vi "III_V_Layer_v23.vi"(2 "Debug Mode":bool, 3 "Elapsed Time(s)":dbl, 4 "State":enum16{"Edit", "Start", "Run", "End", "Idle"}(ring), 5 "Argument List In":string[](array[string])) -> (0 "Status Out":string, 1 "Argument List Out":string[](array[string]))   [LabVIEW 2011]
uses:
  high_level_proc/source_dilution.ctl
  high_level_proc/source_noDilution.ctl
panel:
  in  "run_time":dbl caption="Run Time (s)"
  in  "total_time":dbl
  in  "Ring":u16(ring)
  out "source array":refnum<vi>[](array[refnum])
  in  "Zn_bubbler":T1={"Dilution"=FALSE, "Calculated"=0, "MFC1 flow"=0.0, "MFC2 flow"=10.0, "MFC3 flow"=100.0, "Main"={"Flow"=0.0, "Prep"=FALSE, "Run"=FALSE, "Active"=FALSE, "Name"="Zn"}} caption="Al" {"Main"."Flow" format="%.2f"; "MFC1 flow" format="%.4f"; "MFC3 flow" format="%.1f"; "MFC2 flow" format="%.2f"; "Calculated" items=["Flow", "MFC1", "MFC2", "MFC3"]}
  in  "Al_bubbler":T2={"Flow"=0.0, "Prep"=FALSE, "Run"=FALSE, "Active"=FALSE, "Name"="Al"} caption="Al" {"Flow" format="%.2f"}
  in  "Se_bubbler":T1={"Dilution"=FALSE, "Calculated"=0, "MFC1 flow"=0.0, "MFC2 flow"=10.0, "MFC3 flow"=100.0, "Main"={"Flow"=0.0, "Prep"=FALSE, "Run"=FALSE, "Active"=FALSE, "Name"="Se"}} caption="Al" {"Main"."Flow" format="%.2f"; "MFC1 flow" format="%.4f"; "MFC3 flow" format="%.1f"; "MFC2 flow" format="%.2f"; "Calculated" items=["Flow", "MFC1", "MFC2", "MFC3"]}
  in  "P_bubbler":T2={"Flow"=0.0, "Prep"=FALSE, "Run"=FALSE, "Active"=FALSE, "Name"="P liq"} caption="Al" {"Flow" format="%.2f"}
  in  "As_gas":T2={"Flow"=0.0, "Prep"=FALSE, "Run"=FALSE, "Active"=FALSE, "Name"="As gas"} caption="Al" {"Flow" format="%.2f"}
  in  "P_gas":T2={"Flow"=0.0, "Prep"=FALSE, "Run"=FALSE, "Active"=FALSE, "Name"="P gas"} caption="Al" {"Flow" format="%.2f"}
  in  "In_bubbler":T2={"Flow"=0.0, "Prep"=FALSE, "Run"=FALSE, "Active"=FALSE, "Name"="In"} caption="Al" {"Flow" format="%.2f"}
  in  "Ga_bubbler":T1={"Dilution"=FALSE, "Calculated"=0, "MFC1 flow"=0.0, "MFC2 flow"=10.0, "MFC3 flow"=100.0, "Main"={"Flow"=0.0, "Prep"=FALSE, "Run"=FALSE, "Active"=FALSE, "Name"="Ga"}} caption="Al" {"Main"."Flow" format="%.2f"; "MFC1 flow" format="%.4f"; "MFC3 flow" format="%.1f"; "MFC2 flow" format="%.2f"; "Calculated" items=["Flow", "MFC1", "MFC2", "MFC3"]}
  out "prep_done":bool
  out "run started":bool
  out "first":bool=TRUE
  out "is OK?":bool
  in  "prep_time":dbl caption="Pre-Run Time (s)"
  in  "Cancel":bool
  in  "OK":bool
  # "s"
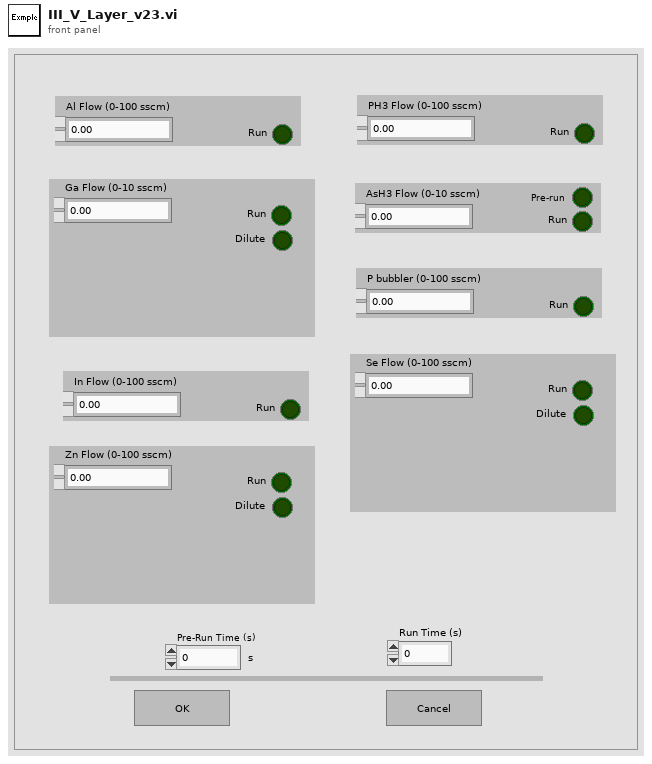
[diagram p1: front panel]
types:
  T1 = typedef "source_dilution.ctl" = cluster{"Dilution":bool, "Calculated":u16, "MFC1 flow":dbl, "MFC2 flow":dbl, "MFC3 flow":dbl, "Main":T2}
  T2 = typedef "source_noDilution.ctl" = cluster{"Flow":dbl, "Prep":bool, "Run":bool, "Active":bool, "Name":string}
  T3 = enum32{"Invalid", "Default", "Floating", "Floating/Auto-Hide", "Modal"}
  T4 = enum16{"Discrete", "Continuous", "Instantaneous", "Finite"}
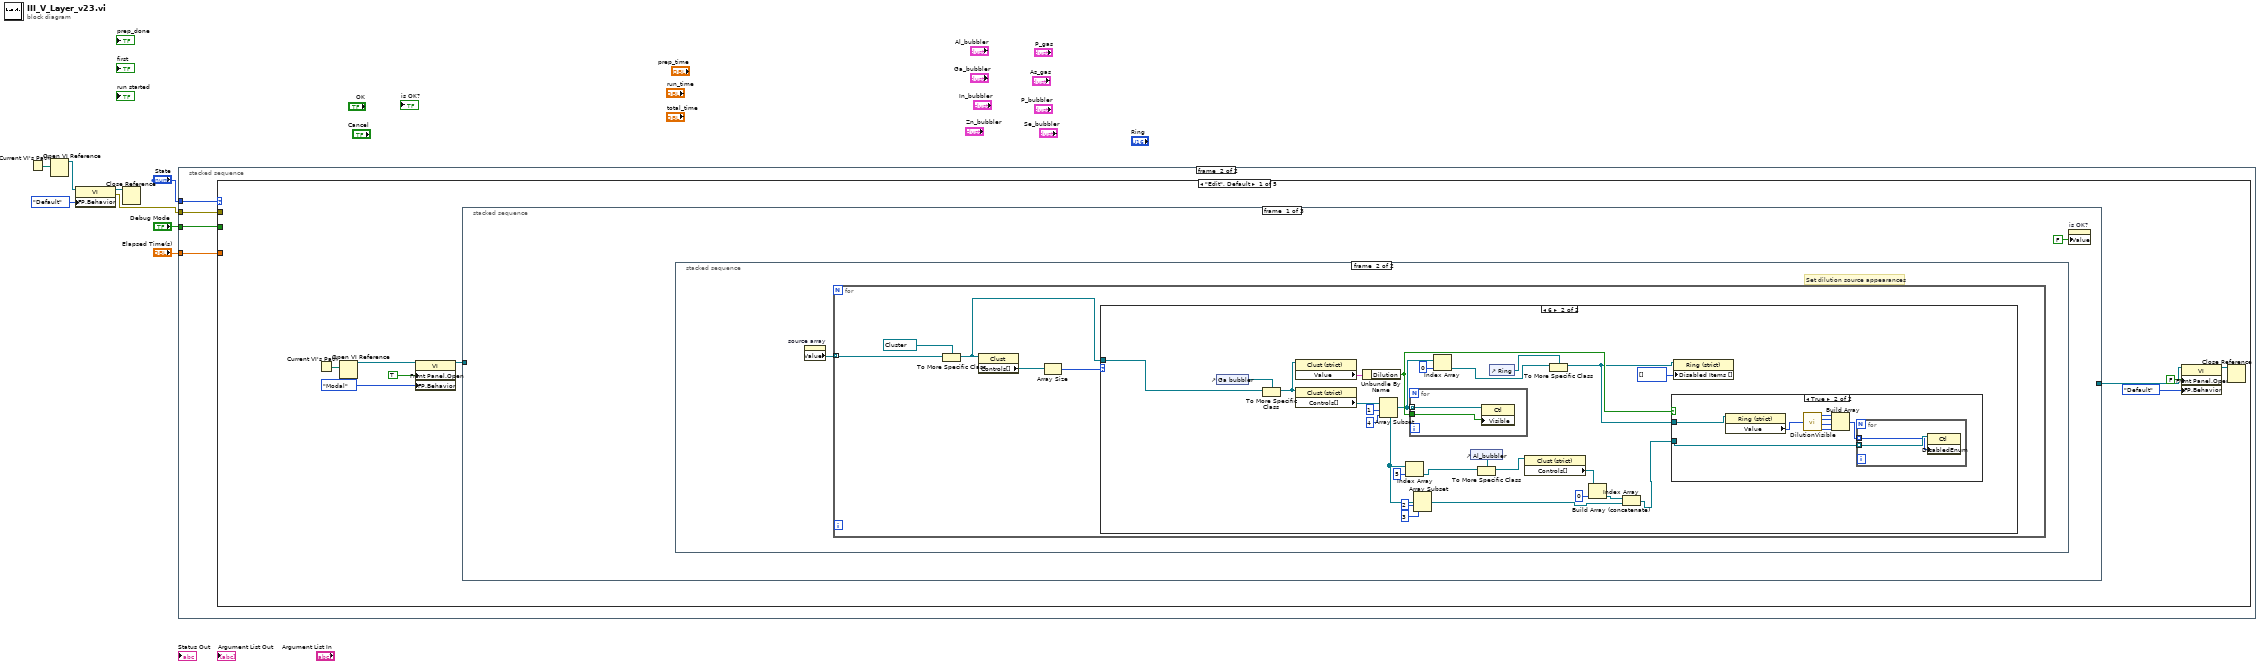
[diagram p0: block diagram]
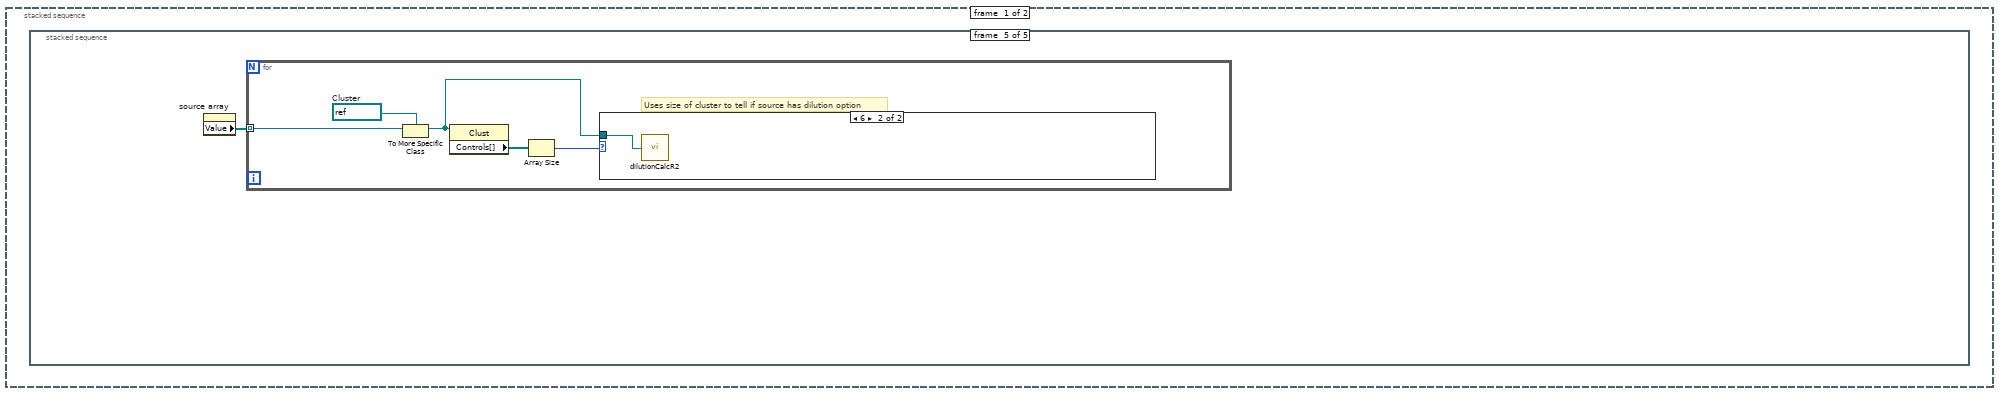
[diagram p2: hidden frame]
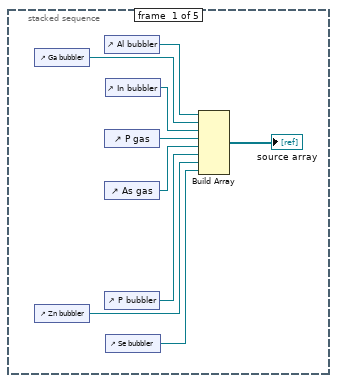
[diagram p3: hidden frame]
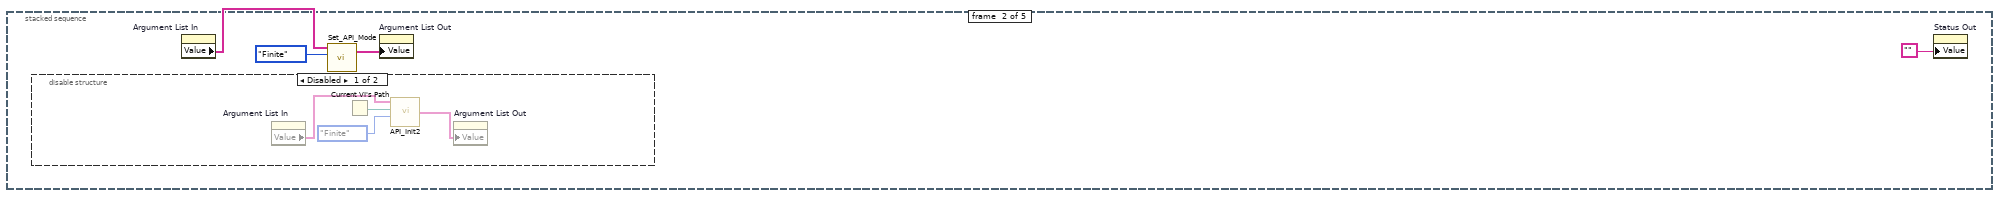
[diagram p4: hidden frame]
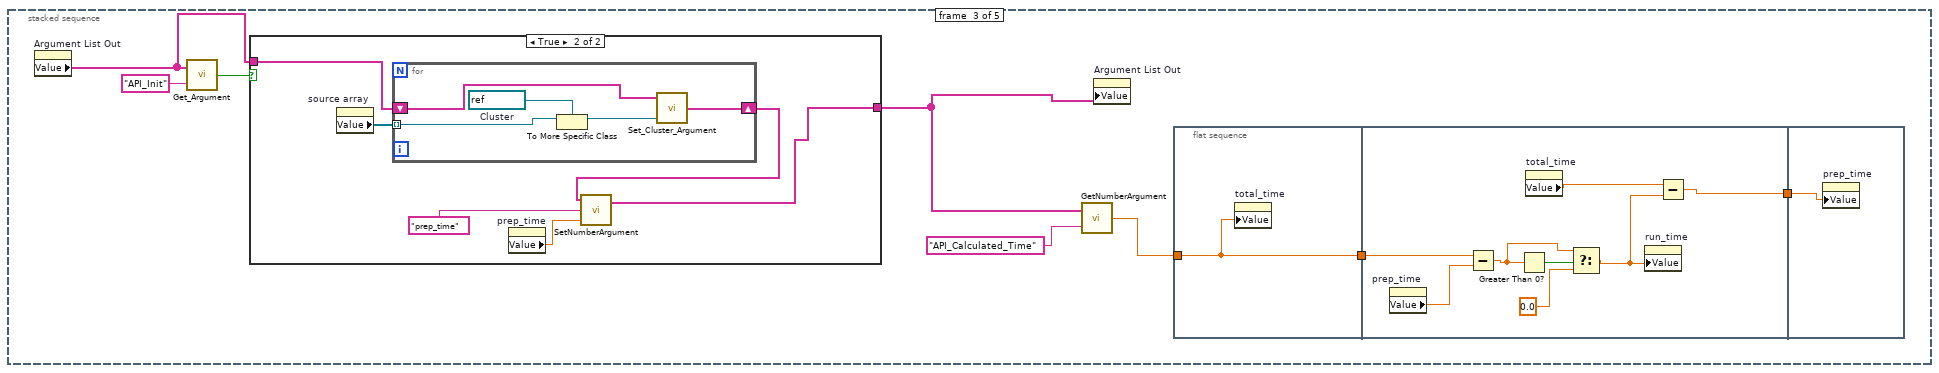
[diagram p6: hidden frame]
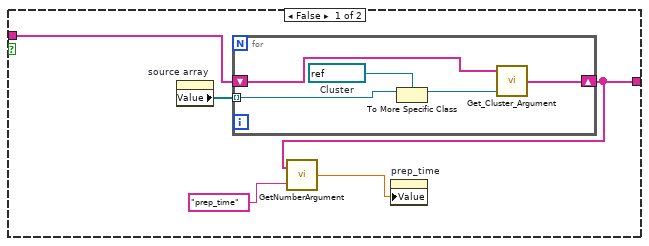
[diagram p7: hidden frame]
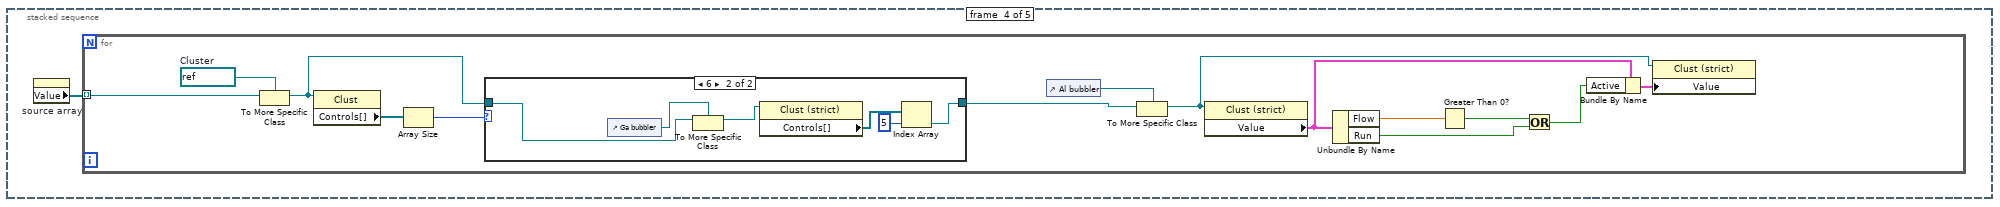
[diagram p8: hidden frame]
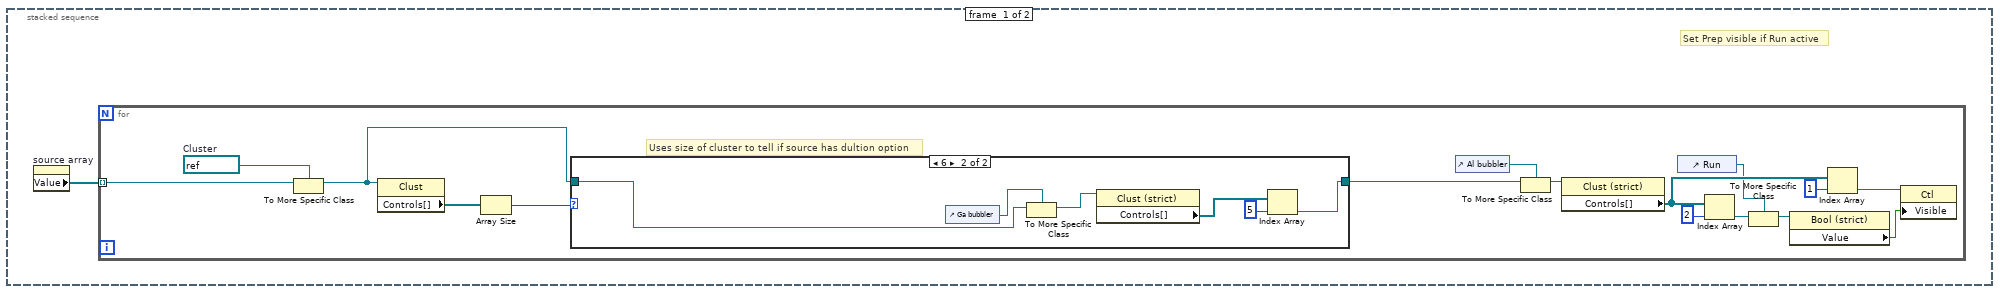
[diagram p11: hidden frame]
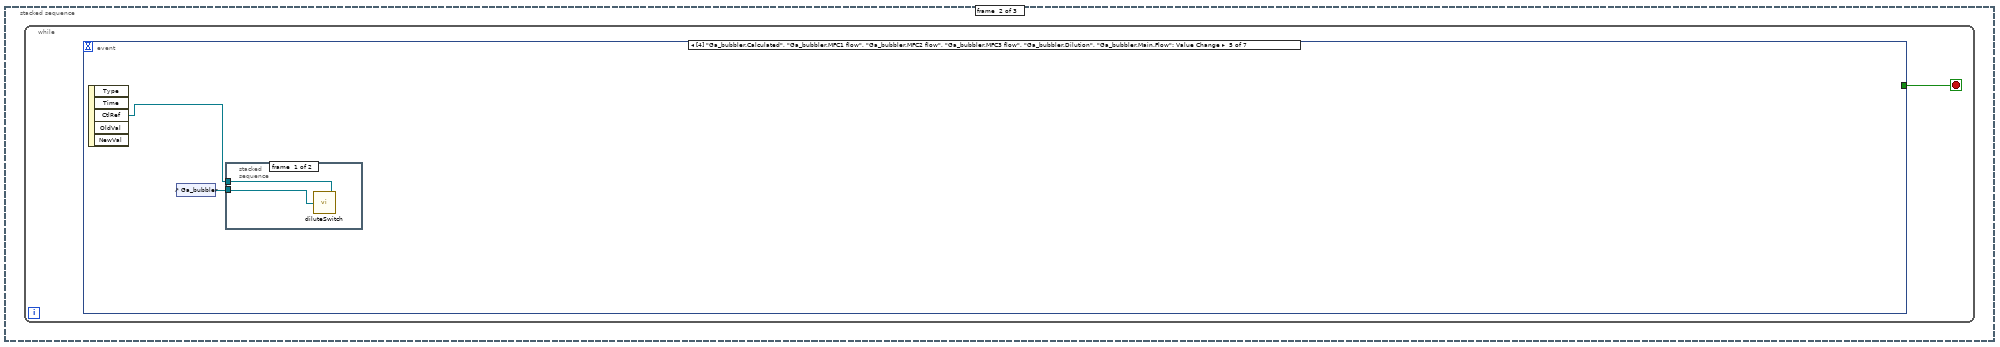
[diagram p15: hidden frame]
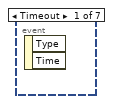
[diagram p16: hidden frame]
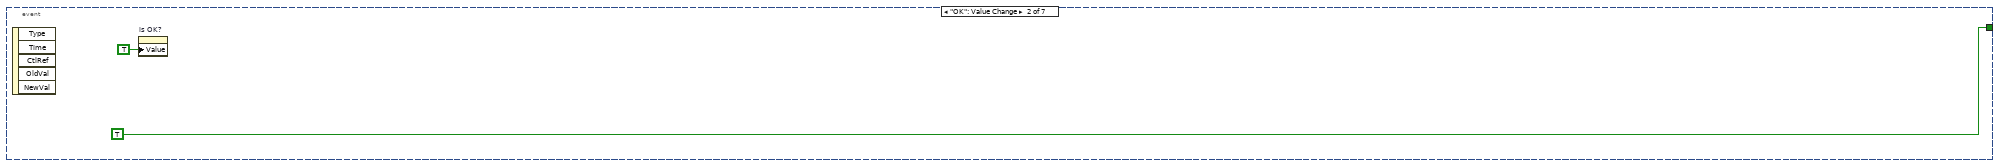
[diagram p17: hidden frame]
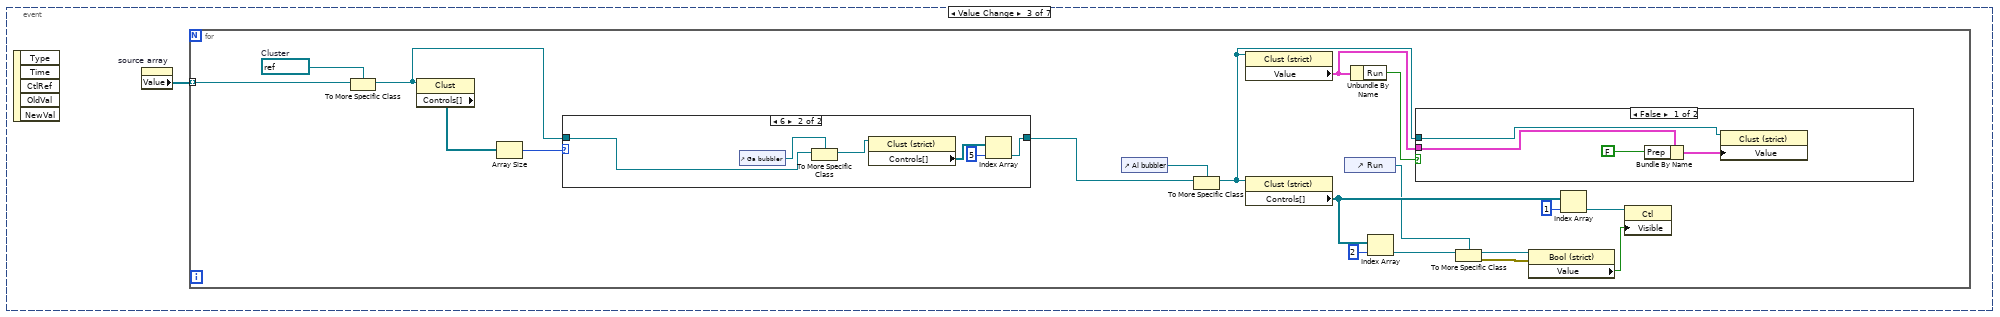
[diagram p18: hidden frame]
diagram:
  n1 = Current VI's Path() -> (path=w5:path)
  n2 = Open VI Reference(vi path=w5) -> (vi reference=w4:refnum<vi>)  [unwired: 1 in, 5 out]
  n3 = property class="VI"(reference=w4, "FP.Behavior"=T3."Default" ("Front Panel Window:Behavior")) -> (reference out=w2:refnum<vi>, error out=w1:errorcluster)  [unwired: 1 in]
  n4 = Close Reference(reference=w2) -> ()  [unwired: 1 in, 1 out]
  n5 = stacked-sequence {
    tunnel: "State" -> [_ w97]
    tunnel: "Debug Mode" -> [_ w96]
    tunnel: "Elapsed Time(s)" -> [_ w95]
    tunnel: w1 -> [_ w94]
    frame #0 {
      n6 = stacked-sequence {
        frame #0 {
          n7 = control-ref of="Ga bubbler"() -> (w12:refnum<vi>)
          n8 = control-ref of="Zn bubbler"() -> (w11:refnum<vi>)
          n9 = control-ref of="Al bubbler"() -> (w17:refnum<vi>)
          n10 = control-ref of="P gas"() -> (w15:refnum<vi>)
          n11 = control-ref of="As gas"() -> (w14:refnum<vi>)
          n12 = control-ref of="P bubbler"() -> (w13:refnum<vi>)
          n13 = control-ref of="In bubbler"() -> (w16:refnum<vi>)
          n14 = control-ref of="Se bubbler"() -> (w10:refnum<vi>)
          n15 = Build Array(w17, w12, w16, w15, w14, w13, w11, w10) -> (→"source array":refnum<vi>[])
        }
        frame #1 {
          n16 = disable-structure shown="Disabled" {
            frame Disabled {
              n17 = property on="Argument List In" class="Arr (strict)"() -> ("Value"=w25:string[])  [unwired: 2 in, 2 out]
              n18 = Current VI's Path() -> (path=w22:path)
              n19 = call "API_Init2.vi"("API Mode"=T4."Finite", "VI Path"=w22, "Argument List In"=w25) -> ("Argument List Out"=w24:string[])  [unwired: 1 in]
              n20 = property on="Argument List Out" class="Arr (strict)"("Value"=w24) -> ()  [unwired: 2 in, 2 out]
            }
            frame Enabled {
            }
          }
          n21 = property on="Argument List In" class="Arr (strict)"() -> ("Value"=w20:string[])  [unwired: 2 in, 2 out]
          n22 = call "Set_API_Mode.vi"("API Mode"=T4."Finite", "Argument List In"=w20) -> ("Argument List Out"=w18:string[])  [unwired: 3 in]
          n23 = property on="Argument List Out" class="Arr (strict)"("Value"=w18) -> ()  [unwired: 2 in, 2 out]
          n24 = property on="Status Out" class="Str"("Value"="") -> ()  [unwired: 2 in, 2 out]
        }
        frame #2 {
          n25 = property on="Argument List Out" class="Arr (strict)"() -> ("Value"=w31:string[])  [unwired: 2 in, 2 out]
          n26 = call "Get_Argument.vi"("Argument"="API_Init", "Argument List"=w31) -> ("Enabled"=w32:bool)
          n27 = case shown="True" w32 {
            tunnel: w31 -> [w48 w59]
            tunnel: [w44 w54] -> w29
            frame False {
              n28 = property on="source array" class="Arr (strict)"() -> ("Value"=w47:refnum<vi>[])  [unwired: 2 in, 2 out]
              n29 = for {
                shift-right: [w52] -> w44
                shift-left: w48 -> [w53]
                tunnel: w47 -> [w51] mode=indexing
                w49 = refnum<vi> refnum  # Cluster
                n30 = To More Specific Class(target class=w49, reference=w51) -> (specific class reference=w50:refnum<vi>)  [unwired: 1 in, 1 out]
                n31 = call "Get_Cluster_Argument.vi"("source"=w50, "Argument List In"=w53) -> ("Argument List Out"=w52:string[])  [unwired: 1 in]
              }
              n32 = call "GetNumberArgument.vi"("Argument"="prep_time", "Argument List In"=w44) -> ("value"=w45:dbl)
              n33 = property on="prep_time" class="DigNum (strict)"("Value"=w45) -> ()  [unwired: 2 in, 2 out]
            }
            frame True {
              n34 = property on="source array" class="Arr (strict)"() -> ("Value"=w58:refnum<vi>[])  [unwired: 2 in, 2 out]
              n35 = for {
                shift-right: [w63] -> w56
                shift-left: w59 -> [w64]
                tunnel: w58 -> [w62] mode=indexing
                w61 = refnum<vi> refnum  # Cluster
                n36 = To More Specific Class(target class=w61, reference=w62) -> (specific class reference=w60:refnum<vi>)  [unwired: 1 in, 1 out]
                n37 = call "Set_Cluster_Argument.vi"("Clust Refnum"=w60, "Argument List In"=w64) -> ("Argument List Out"=w63:string[])  [unwired: 1 in]
              }
              n38 = property on="prep_time" class="DigNum (strict)"() -> ("Value"=w55:dbl)  [unwired: 2 in, 2 out]
              n39 = call "SetNumberArgument.vi"("value"=w55, "Argument"="prep_time", "Argument List In"=w56) -> ("Argument List Out"=w54:string[])  [unwired: 1 out]
            }
          }
          n40 = call "GetNumberArgument.vi"("Argument"="API_Calculated_Time", "Argument List In"=w29) -> ("value"=w28:dbl)
          n41 = property on="Argument List Out" class="Arr (strict)"("Value"=w29) -> ()  [unwired: 2 in, 2 out]
          n42 = flat-sequence {
            tunnel: w28 -> [w34]
            tunnel: [w34] -> w27
            tunnel: w27 -> [w38]
            tunnel: [w35] -> w26
            tunnel: w26 -> [w43]
            frame #0 {
              n43 = property on="total_time" class="DigNum (strict)"("Value"=w34) -> ()  [unwired: 2 in, 2 out]
            }
            frame #1 {
              n44 = property on="prep_time" class="DigNum (strict)"() -> ("Value"=w42:dbl)  [unwired: 2 in, 2 out]
              n45 = Subtract(x=w38, y=w42) -> (x-y=w39:dbl)
              n46 = Greater Than 0?(x=w39) -> (x > 0?=w40:bool)
              n47 = property on="total_time" class="DigNum (strict)"() -> ("Value"=w37:dbl)  [unwired: 2 in, 2 out]
              n48 = Select(t=w39, s=w40, f=0.0) -> (s? t:f=w36:dbl)
              n49 = property on="run_time" class="DigNum (strict)"("Value"=w36) -> ()  [unwired: 2 in, 2 out]
              n50 = Subtract(x=w37, y=w36) -> (x-y=w35:dbl)
            }
            frame #2 {
              n51 = property on="prep_time" class="DigNum (strict)"("Value"=w43) -> ()  [unwired: 2 in, 2 out]
            }
          }
        }
        frame #3 {
          n52 = property on="source array" class="Arr (strict)"() -> ("Value"=w65:refnum<vi>[])  [unwired: 2 in, 2 out]
          n53 = for {
            tunnel: w65 -> [w68] mode=indexing
            w66 = refnum<vi> refnum  # Cluster
            n54 = To More Specific Class(target class=w66, reference=w68) -> (specific class reference=w67:refnum<vi>)  [unwired: 1 in, 1 out]
            n55 = property class="Clust"(reference=w67) -> ("Controls[]"=w70:refnum<vi>[])  [unwired: 1 in, 2 out]
            n56 = Array Size(array=w70) -> (size(s)=w71:i32)
            n57 = case shown="6" w71 {
              tunnel: [w80 w82] -> w69
              tunnel: w67 -> [w80 w85]
              frame Default {
              }
              frame 6 {
                n58 = control-ref of="Ga bubbler"() -> (w81:refnum<vi>)
                n59 = To More Specific Class(target class=w81, reference=w85) -> (specific class reference=w84:refnum<vi>)  [unwired: 1 in, 1 out]
                n60 = property class="Clust (strict)"(reference=w84) -> ("Controls[]"=w83:refnum<vi>[])  [unwired: 1 in, 2 out]
                n61 = Index Array(array=w83, index=5) -> (element=w82:refnum<vi>)
              }
            }
            n62 = control-ref of="Al bubbler"() -> (w73:refnum<vi>)
            n63 = To More Specific Class(target class=w73, reference=w69) -> (specific class reference=w72:refnum<vi>)  [unwired: 1 in, 1 out]
            n64 = property class="Clust (strict)"(reference=w72) -> ("Value"=w76:T2)  [unwired: 1 in, 2 out]
            n65 = Unbundle By Name(w76) -> ("Flow"=w79:dbl, "Run"=w77:bool)
            n66 = Greater Than 0?(x=w79) -> (x > 0?=w78:bool)
            n67 = Or(x=w78, y=w77) -> (x .or. y?=w74:bool)
            n68 = Bundle By Name(cluster=w76, "Active"=w74) -> (w75:T2)
            n69 = property class="Clust (strict)"(reference=w72, "Value"=w75) -> ()  [unwired: 1 in, 2 out]
          }
        }
        frame #4 {
          n70 = property on="source array" class="Arr (strict)"() -> ("Value"=w87:refnum<vi>[])  [unwired: 2 in, 2 out]
          n71 = for {
            tunnel: w87 -> [w91] mode=indexing
            w89 = refnum<vi> refnum  # Cluster
            # "Uses size of cluster to tell if source has dilution option"
            n72 = To More Specific Class(target class=w89, reference=w91) -> (specific class reference=w90:refnum<vi>)  [unwired: 1 in, 1 out]
            n73 = property class="Clust"(reference=w90) -> ("Controls[]"=w88:refnum<vi>[])  [unwired: 1 in, 2 out]
            n74 = Array Size(array=w88) -> (size(s)=w92:i32)
            n75 = case shown="6" w92 {
              tunnel: w90 -> [_ w93]
              frame Default {
              }
              frame 6 {
                n76 = call "dilutionCalcR2.vi"("Clust Refnum"=w93) -> ()
              }
            }
          }
        }
      }
    }
    frame #1 {
      n77 = case shown="\"Edit\", Default" w97 {
        tunnel: w96 -> [_ w251 w267 _ _]
        tunnel: w95 -> [_ _ w268 _ _]
        tunnel: w94 -> [_ _ _ _ _]
        frame "Edit", Default {
          n78 = Current VI's Path() -> (path=w102:path)
          n79 = Open VI Reference(vi path=w102) -> (vi reference=w101:refnum<vi>)  [unwired: 1 in, 5 out]
          n80 = property class="VI"(reference=w101, "Front Panel.Open"=TRUE ("Front Panel Window:Open"), "FP.Behavior"=T3."Modal" ("Front Panel Window:Behavior")) -> (reference out=w99:refnum<vi>)  [unwired: 1 in, 1 out]
          n81 = stacked-sequence {
            tunnel: [_ _ w227] -> w104
            tunnel: w99 -> [_ _ w227]
            frame #0 {
              n82 = stacked-sequence {
                frame #0 {
                  # "Set Prep visible if Run active"
                  n83 = property on="source array" class="Arr (strict)"() -> ("Value"=w108:refnum<vi>[])  [unwired: 2 in, 2 out]
                  n84 = for {
                    tunnel: w108 -> [w113] mode=indexing
                    w112 = refnum<vi> refnum  # Cluster
                    # "Uses size of cluster to tell if source has dultion option"
                    n85 = To More Specific Class(target class=w112, reference=w113) -> (specific class reference=w109:refnum<vi>)  [unwired: 1 in, 1 out]
                    n86 = property class="Clust"(reference=w109) -> ("Controls[]"=w111:refnum<vi>[])  [unwired: 1 in, 2 out]
                    n87 = Array Size(array=w111) -> (size(s)=w110:i32)
                    n88 = case shown="6" w110 {
                      tunnel: w109 -> [w125 w128]
                      tunnel: [w125 w129] -> w115
                      frame Default {
                      }
                      frame 6 {
                        n89 = control-ref of="Ga bubbler"() -> (w126:refnum<vi>)
                        n90 = To More Specific Class(target class=w126, reference=w128) -> (specific class reference=w127:refnum<vi>)  [unwired: 1 in, 1 out]
                        n91 = property class="Clust (strict)"(reference=w127) -> ("Controls[]"=w131:refnum<vi>[])  [unwired: 1 in, 2 out]
                        n92 = Index Array(array=w131, index=5) -> (element=w129:refnum<vi>)
                      }
                    }
                    n93 = control-ref of="Al bubbler"() -> (w116:refnum<vi>)
                    n94 = To More Specific Class(target class=w116, reference=w115) -> (specific class reference=w122:refnum<vi>)  [unwired: 1 in, 1 out]
                    n95 = property class="Clust (strict)"(reference=w122) -> ("Controls[]"=w121:refnum<vi>[])  [unwired: 1 in, 2 out]
                    n96 = control-ref of="Run"() -> (w114:refnum<vi>)
                    n97 = Index Array(array=w121, index=2) -> (element=w119:refnum<vi>)
                    n98 = To More Specific Class(target class=w114, reference=w119) -> (specific class reference=w118:refnum<vi>)  [unwired: 1 in, 1 out]
                    n99 = property class="Bool (strict)"(reference=w118) -> ("Value"=w117:bool)  [unwired: 1 in, 2 out]
                    n100 = Index Array(array=w121, index=1) -> (element=w123:refnum<vi>)
                    n101 = property class="Ctl"(reference=w123, "Visible"=w117) -> ()  [unwired: 1 in, 2 out]
                  }
                }
                frame #1 {
                  # "Set dilution source appearances"
                  n102 = property on="source array" class="Arr (strict)"() -> ("Value"=w132:refnum<vi>[])  [unwired: 2 in, 2 out]
                  n103 = for {
                    tunnel: w132 -> [w137] mode=indexing
                    n104 = To More Specific Class(target class=refnum<vi> refnum, reference=w137) -> (specific class reference=w133:refnum<vi>)  [unwired: 1 in, 1 out]
                    n105 = property class="Clust"(reference=w133) -> ("Controls[]"=w135:refnum<vi>[])  [unwired: 1 in, 2 out]
                    n106 = Array Size(array=w135) -> (size(s)=w134:i32)
                    n107 = case shown="6" w134 {
                      tunnel: w133 -> [_ w162]
                      frame Default {
                      }
                      frame 6 {
                        n108 = control-ref of="Ga bubbler"() -> (w161:refnum<vi>)
                        n109 = To More Specific Class(target class=w161, reference=w162) -> (specific class reference=w159:refnum<vi>)  [unwired: 1 in, 1 out]
                        n110 = property class="Clust (strict)"(reference=w159) -> ("Value"=w160:T1)  [unwired: 1 in, 2 out]
                        n111 = property class="Clust (strict)"(reference=w159) -> ("Controls[]"=w147:refnum<vi>[])  [unwired: 1 in, 2 out]
                        n112 = Unbundle By Name(w160) -> ("Dilution"=w153:bool)
                        n113 = Array Subset(array=w147, index=1, length=4) -> (w151:refnum<vi>[])
                        n114 = Index Array(array=w147, index=5) -> (element=w145:refnum<vi>)
                        n115 = for {
                          tunnel: w151 -> [w174] mode=indexing
                          tunnel: w153 -> [w173]
                          n116 = property class="Ctl"(reference=w174, "Visible"=w173) -> ()  [unwired: 1 in, 2 out]
                        }
                        n117 = Array Subset(array=w147, index=2, length=3) -> (w139:refnum<vi>[])
                        n118 = Index Array(array=w151, index=0) -> (element=w152:refnum<vi>)
                        n119 = control-ref of="Al_bubbler"() -> (w144:refnum<vi>)
                        n120 = To More Specific Class(target class=w144, reference=w145) -> (specific class reference=w143:refnum<vi>)  [unwired: 1 in, 1 out]
                        n121 = control-ref of="Ring"() -> (w155:refnum<vi>)
                        n122 = property class="Clust (strict)"(reference=w143) -> ("Controls[]"=w142:refnum<vi>[])  [unwired: 1 in, 2 out]
                        n123 = To More Specific Class(target class=w155, reference=w152) -> (specific class reference=w150:refnum<vi>)  [unwired: 1 in, 1 out]
                        n124 = Index Array(array=w142, index=0) -> (element=w140:refnum<vi>)
                        n125 = Build Array (concatenate)(w140, w139) -> (w138:refnum<vi>[])
                        n126 = case shown="True" w153 {
                          tunnel: w150 -> [_ w163]
                          tunnel: w138 -> [_ w165]
                          frame False {
                          }
                          frame True {
                            n127 = property class="Ring (strict)"(reference=w163) -> ("Value"=w164:u16)  [unwired: 1 in, 2 out]
                            n128 = call "DilutionVisible.vi"("calculated"=w164) -> ("flow"=w170:u16, "MFC1"=w169:u16, "MFC2"=w168:u16, "MFC3"=w167:u16)
                            n129 = Build Array(w170, w169, w168, w167) -> (w166:u16[])
                            n130 = for {
                              tunnel: w166 -> [w171] mode=indexing
                              tunnel: w165 -> [w172] mode=indexing
                              n131 = property class="Ctl"(reference=w172, "DisabledEnum"=w171) -> ()  [unwired: 1 in, 2 out]
                            }
                          }
                        }
                        n132 = property class="Ring (strict)"(reference=w150, "Disabled Items []"=i32[] []) -> ()  [unwired: 1 in, 2 out]
                      }
                    }
                  }
                }
              }
              n133 = property on="is OK?" class="Bool (strict)"("Value"=FALSE ("is OK?")) -> ()  [unwired: 2 in, 2 out]
            }
            frame #1 {
              n134 = while {
                stop <- w175 stop-if-true
                n135 = event shown="[4] \"Ga_bubbler.Calculated\", \"Ga_bubbler.MFC1 flow\", \"Ga_bubbler.MFC2 flow\", \"Ga_bubbler.MFC3 flow\", \"Ga_bubbler.Dilution\", \"Ga_bubbler.Main.Flow\": Value Change" {
                  selector: _ -> [_ _ _ _ _ _ _]
                  dyn-events: _ -> [_ _ _ _ _ _ _]
                  timeout: _ -> [_ _ _ _ _ _ _]
                  tunnel: [_ TRUE _ TRUE _ _ _] -> w175
                  event Timeout {
                    n136 = event-data() -> ()  [unwired: 1 in, 2 out]
                  }
                  event "OK": Value Change {
                    n137 = event-data() -> ()  [unwired: 1 in, 5 out]
                    n138 = property on="is OK?" class="Bool (strict)"("Value"=TRUE ("is OK?")) -> ()  [unwired: 2 in, 2 out]
                  }
                  event Value Change {
                    n139 = event-data() -> ()  [unwired: 1 in, 5 out]
                    n140 = property on="source array" class="Arr (strict)"() -> ("Value"=w178:refnum<vi>[])  [unwired: 2 in, 2 out]
                    n141 = for {
                      tunnel: w178 -> [w181] mode=indexing
                      w179 = refnum<vi> refnum  # Cluster
                      n142 = To More Specific Class(target class=w179, reference=w181) -> (specific class reference=w180:refnum<vi>)  [unwired: 1 in, 1 out]
                      n143 = property class="Clust"(reference=w180) -> ("Controls[]"=w183:refnum<vi>[])  [unwired: 1 in, 2 out]
                      n144 = Array Size(array=w183) -> (size(s)=w182:i32)
                      n145 = case shown="6" w182 {
                        tunnel: w180 -> [w198 w201]
                        tunnel: [w198 w202] -> w185
                        frame Default {
                        }
                        frame 6 {
                          n146 = control-ref of="Ga bubbler"() -> (w199:refnum<vi>)
                          n147 = To More Specific Class(target class=w199, reference=w201) -> (specific class reference=w200:refnum<vi>)  [unwired: 1 in, 1 out]
                          n148 = property class="Clust (strict)"(reference=w200) -> ("Controls[]"=w204:refnum<vi>[])  [unwired: 1 in, 2 out]
                          n149 = Index Array(array=w204, index=5) -> (element=w202:refnum<vi>)
                        }
                      }
                      n150 = control-ref of="Al bubbler"() -> (w189:refnum<vi>)
                      n151 = To More Specific Class(target class=w189, reference=w185) -> (specific class reference=w186:refnum<vi>)  [unwired: 1 in, 1 out]
                      n152 = property class="Clust (strict)"(reference=w186) -> ("Value"=w188:T2)  [unwired: 1 in, 2 out]
                      n153 = property class="Clust (strict)"(reference=w186) -> ("Controls[]"=w195:refnum<vi>[])  [unwired: 1 in, 2 out]
                      n154 = control-ref of="Run"() -> (w184:refnum<vi>)
                      n155 = Unbundle By Name(w188) -> ("Run"=w187:bool)
                      n156 = Index Array(array=w195, index=2) -> (element=w193:refnum<vi>)
                      n157 = case shown="False" w187 {
                        tunnel: w188 -> [w208 _]
                        tunnel: w186 -> [w205 _]
                        frame False {
                          n158 = Bundle By Name(cluster=w208, "Prep"=FALSE) -> (w206:T2)
                          n159 = property class="Clust (strict)"(reference=w205, "Value"=w206) -> ()  [unwired: 1 in, 2 out]
                        }
                        frame True {
                        }
                      }
                      n160 = To More Specific Class(target class=w184, reference=w193) -> (specific class reference=w192:refnum<vi>, error out=w191:errorcluster)  [unwired: 1 in]
                      n161 = property class="Bool (strict)"(reference=w192, error in=w191) -> ("Value"=w190:bool)  [unwired: 2 out]
                      n162 = Index Array(array=w195, index=1) -> (element=w196:refnum<vi>)
                      n163 = property class="Ctl"(reference=w196, "Visible"=w190) -> ()  [unwired: 1 in, 2 out]
                    }
                  }
                  event "Cancel": Value Change {
                    n164 = event-data() -> ()  [unwired: 1 in, 5 out]
                  }
                  event Value Change {
                    n165 = event-data() -> ("CtlRef"=w210:refnum<vi>)  [unwired: 1 in, 4 out]
                    n166 = control-ref of="Ga_bubbler"() -> (w211:refnum<vi>)
                    n167 = stacked-sequence {
                      tunnel: w211 -> [w213 w214]
                      tunnel: w210 -> [w212 _]
                      frame #0 {
                        n168 = call "diluteSwitch.vi"("Ctl Refnum"=w212, "Clust Refnum"=w213) -> ()
                      }
                      frame #1 {
                        n169 = call "dilutionCalcR2.vi"("Clust Refnum"=w214) -> ()
                      }
                    }
                  }
                  event Value Change {
                    n170 = event-data() -> ("CtlRef"=w215:refnum<vi>)  [unwired: 1 in, 4 out]
                    n171 = control-ref of="Zn_bubbler"() -> (w216:refnum<vi>)
                    n172 = stacked-sequence {
                      tunnel: w216 -> [w218 w219]
                      tunnel: w215 -> [w217 _]
                      frame #0 {
                        n173 = call "diluteSwitch.vi"("Ctl Refnum"=w217, "Clust Refnum"=w218) -> ()
                      }
                      frame #1 {
                        n174 = call "dilutionCalcR2.vi"("Clust Refnum"=w219) -> ()
                      }
                    }
                  }
                  event Value Change {
                    n175 = event-data() -> ("CtlRef"=w220:refnum<vi>)  [unwired: 1 in, 4 out]
                    n176 = control-ref of="Se_bubbler"() -> (w221:refnum<vi>)
                    n177 = stacked-sequence {
                      tunnel: w221 -> [w223 w224]
                      tunnel: w220 -> [w222 _]
                      frame #0 {
                        n178 = call "diluteSwitch.vi"("Ctl Refnum"=w222, "Clust Refnum"=w223) -> ()
                      }
                      frame #1 {
                        n179 = call "dilutionCalcR2.vi"("Clust Refnum"=w224) -> ()
                      }
                    }
                  }
                }
              }
            }
            frame #2 {
              n180 = property on="Argument List Out" class="Arr (strict)"() -> ("Value"=w226:string[])  [unwired: 2 in, 2 out]
              n181 = property on="is OK?" class="Bool (strict)"() -> ("Value"=w228:bool)  [unwired: 2 in, 2 out]
              n182 = case shown="True" w228 {
                tunnel: w226 -> [w229 w242]
                tunnel: [w229 w239] -> w225
                frame False {
                }
                frame True {
                  n183 = property on="source array" class="Arr (strict)"() -> ("Value"=w241:refnum<vi>[])  [unwired: 2 in, 2 out]
                  n184 = property on="prep_time" class="DigNum (strict)"() -> ("Value"=w231:dbl)  [unwired: 2 in, 2 out]
                  n185 = for {
                    shift-right: [w246] -> w234
                    shift-left: w242 -> [w247]
                    tunnel: w241 -> [w245] mode=indexing
                    w244 = refnum<vi> refnum  # Cluster
                    n186 = To More Specific Class(target class=w244, reference=w245) -> (specific class reference=w243:refnum<vi>)  [unwired: 1 in, 1 out]
                    n187 = call "Set_Cluster_Argument.vi"("Clust Refnum"=w243, "Argument List In"=w247) -> ("Argument List Out"=w246:string[])  [unwired: 1 in]
                  }
                  n188 = call "SetNumberArgument.vi"("value"=w231, "Argument"="prep_time", "Argument List In"=w234) -> ("Argument List Out"=w235:string[])  [unwired: 1 out]
                  n189 = property on="run_time" class="DigNum (strict)"() -> ("Value"=w232:dbl)  [unwired: 2 in, 2 out]
                  n190 = Add(x=w231, y=w232) -> (x+y=w230:dbl)
                  n191 = call "SetNumberArgument.vi"("value"=w230, "Argument"="API_Calculated_Time", "Argument List In"=w235) -> ("Argument List Out"=w233:string[])  [unwired: 1 out]
                  n192 = call "Set_Argument.vi"("Enable"=FALSE, "Argument"="API_Init", "Argument List In"=w233) -> ("Argument List Out"=w239:string[])
                }
              }
              n193 = property on="Argument List Out" class="Arr (strict)"("Value"=w225) -> ()  [unwired: 2 in, 2 out]
              n194 = property on="is OK?" class="Bool (strict)" props=["Value"]() -> ()  [unwired: 2 in, 3 out]
            }
          }
          n195 = property class="VI"(reference=w104, "Front Panel.Open"=FALSE ("Front Panel Window:Open"), "FP.Behavior"=T3."Default" ("Front Panel Window:Behavior")) -> (reference out=w105:refnum<vi>)  [unwired: 1 in, 1 out]
          n196 = Close Reference(reference=w105) -> ()  [unwired: 1 in, 1 out]
        }
        frame "Start" {
          n197 = property on="prep_time" class="DigNum (strict)"() -> ("Value"=w254:dbl)  [unwired: 2 in, 2 out]
          n198 = Not(x=w251) -> (.not. x?=w250:bool)
          n199 = Greater Than 0?(x=w254) -> (x > 0?=w253:bool)
          n200 = And(x=w250, y=w253) -> (x .and. y?=w252:bool)
          n201 = property on="Argument List Out" class="Arr (strict)"() -> ("Value"=w249:string[])  [unwired: 2 in, 2 out]
          n202 = case shown="True" w252 {
            frame False {
            }
            frame True {
              n203 = property on="Ga_bubbler" class="Clust (strict)"() -> ("Value"=w263:T1)  [unwired: 2 in, 2 out]
              n204 = property on="Zn_bubbler" class="Clust (strict)"() -> ("Value"=w257:T1)  [unwired: 2 in, 2 out]
              n205 = property on="Se_bubbler" class="Clust (strict)"() -> ("Value"=w258:T1)  [unwired: 2 in, 2 out]
              n206 = property on="Al_bubbler" class="Clust (strict)"() -> ("Value"=w264:T2)  [unwired: 2 in, 2 out]
              n207 = property on="P_gas" class="Clust (strict)"() -> ("Value"=w261:T2)  [unwired: 2 in, 2 out]
              n208 = property on="In_bubbler" class="Clust (strict)"() -> ("Value"=w262:T2)  [unwired: 2 in, 2 out]
              n209 = property on="As_gas" class="Clust (strict)"() -> ("Value"=w260:T2)  [unwired: 2 in, 2 out]
              n210 = property on="P_bubbler" class="Clust (strict)"() -> ("Value"=w259:T2)  [unwired: 2 in, 2 out]
              n211 = call "Set_V_III.vi"("Se bubbler"=w258, "P bubbler"=w259, "As gas"=w260, "P gas"=w261, "Run Started"=FALSE, "Zn bubbler"=w257, "In bubbler"=w262, "Ga bubbler"=w263, "Al bubbler"=w264) -> ()  [unwired: 3 in]
            }
          }
          n212 = call "Set_Argument.vi"("Enable"=FALSE, "Argument"="run_started", "Argument List In"=w249) -> ("Argument List Out"=w248:string[])
          n213 = property on="Argument List Out" class="Arr (strict)"("Value"=w248) -> ()  [unwired: 2 in, 2 out]
        }
        frame "Run" {
          n214 = property on="source array" class="Arr (strict)"() -> ("Value"=w266:refnum<vi>[])  [unwired: 2 in, 2 out]
          n215 = stacked-sequence {
            tunnel: w268 -> [_ w273 _ _]
            tunnel: w267 -> [_ _ _ w305]
            tunnel: w266 -> [_ _ w275 _]
            frame #0 {
              n216 = property on="Argument List Out" class="Arr (strict)"() -> ("Value"=w270:string[])  [unwired: 2 in, 2 out]
              n217 = call "Get_Argument.vi"("Argument"="run_started", "Argument List"=w270) -> ("Enabled"=w269:bool)
              n218 = property on="run started" class="Bool (strict)"("Value"=w269) -> ()  [unwired: 2 in, 2 out]
            }
            frame #1 {
              n219 = property on="prep_time" class="DigNum (strict)"() -> ("Value"=w274:dbl)  [unwired: 2 in, 2 out]
              n220 = Greater Or Equal?(x=w273, y=w274) -> (x >= y?=w272:bool)
              n221 = property on="prep_done" class="Bool (strict)"("Value"=w272) -> ()  [unwired: 2 in, 2 out]
            }
            frame #2 {
              n222 = property on="run started" class="Bool (strict)"() -> ("Value"=w276:bool)  [unwired: 2 in, 2 out]
              n223 = Not(x=w276) -> (.not. x?=w278:bool)
              n224 = for {
                shift-right: [w290] -> _
                shift-left: TRUE ("first") -> [w288]
                tunnel: w278 -> [w289]
                tunnel: w275 -> [w282] mode=indexing
                w281 = refnum<vi> refnum  # Cluster
                n225 = To More Specific Class(target class=w281, reference=w282) -> (specific class reference=w280:refnum<vi>)  [unwired: 1 in, 1 out]
                n226 = property class="Clust"(reference=w280) -> ("Controls[]"=w284:refnum<vi>[])  [unwired: 1 in, 2 out]
                n227 = Array Size(array=w284) -> (size(s)=w283:i32)
                n228 = case shown="6" w283 {
                  tunnel: [w297 w300] -> w286
                  tunnel: w280 -> [w297 w298]
                  frame Default {
                  }
                  frame 6 {
                    n229 = control-ref of="Ga bubbler"() -> (w299:refnum<vi>)
                    n230 = To More Specific Class(target class=w299, reference=w298) -> (specific class reference=w303:refnum<vi>)  [unwired: 1 in, 1 out]
                    n231 = property class="Clust (strict)"(reference=w303) -> ("Controls[]"=w302:refnum<vi>[])  [unwired: 1 in, 2 out]
                    n232 = Index Array(array=w302, index=5) -> (element=w300:refnum<vi>)
                  }
                }
                n233 = control-ref of="Al bubbler"() -> (w287:refnum<vi>)
                n234 = To More Specific Class(target class=w287, reference=w286) -> (specific class reference=w285:refnum<vi>)  [unwired: 1 in, 1 out]
                n235 = property class="Clust (strict)"(reference=w285) -> ("Value"=w296:T2)  [unwired: 1 in, 2 out]
                n236 = Unbundle By Name(w296) -> ("Prep"=w295:bool, "Run"=w294:bool, "Active"=w293:bool, "Name"=w279:string)
                n237 = property on="Status Out" class="Str"() -> ("Value"=w292:string)  [unwired: 2 in, 2 out]
                n238 = call "flow_strings.vi"("string in"=w292, "is first in?"=w288, "use source?"=w293, "name"=w279, "run source?"=w294, "prep source?"=w295, "is prep?"=w289) -> ("string out"=w291:string, "is first out?"=w290:bool)
                n239 = property on="Status Out" class="Str"("Value"=w291) -> ()  [unwired: 2 in, 2 out]
              }
            }
            frame #3 {
              n240 = property on="run started" class="Bool (strict)"() -> ("Value"=w307:bool)  [unwired: 2 in, 2 out]
              n241 = Not(x=w307) -> (.not. x?=w306:bool)
              n242 = property on="prep_done" class="Bool (strict)"() -> ("Value"=w308:bool)  [unwired: 2 in, 2 out]
              n243 = And(x=w308, y=w306) -> (x .and. y?=w304:bool)
              n244 = case shown="True" w304 {
                selector: w304 -> [_ w309]
                tunnel: w305 -> [_ w310]
                frame False {
                }
                frame True {
                  n245 = stacked-sequence {
                    tunnel: w310 -> [w312 _]
                    tunnel: w309 -> [w311 _]
                    frame #0 {
                      n246 = case shown="False" w312 {
                        tunnel: w311 -> [w321 _]
                        frame False {
                          n247 = property on="Zn_bubbler" class="Clust (strict)"() -> ("Value"=w313:T1)  [unwired: 2 in, 2 out]
                          n248 = property on="Se_bubbler" class="Clust (strict)"() -> ("Value"=w314:T1)  [unwired: 2 in, 2 out]
                          n249 = property on="Ga_bubbler" class="Clust (strict)"() -> ("Value"=w319:T1)  [unwired: 2 in, 2 out]
                          n250 = property on="Al_bubbler" class="Clust (strict)"() -> ("Value"=w320:T2)  [unwired: 2 in, 2 out]
                          n251 = property on="P_gas" class="Clust (strict)"() -> ("Value"=w317:T2)  [unwired: 2 in, 2 out]
                          n252 = property on="In_bubbler" class="Clust (strict)"() -> ("Value"=w318:T2)  [unwired: 2 in, 2 out]
                          n253 = property on="As_gas" class="Clust (strict)"() -> ("Value"=w316:T2)  [unwired: 2 in, 2 out]
                          n254 = property on="P_bubbler" class="Clust (strict)"() -> ("Value"=w315:T2)  [unwired: 2 in, 2 out]
                          n255 = call "Set_V_III.vi"("Se bubbler"=w314, "P bubbler"=w315, "As gas"=w316, "P gas"=w317, "Run Started"=w321, "Zn bubbler"=w313, "In bubbler"=w318, "Ga bubbler"=w319, "Al bubbler"=w320) -> ()  [unwired: 3 in]
                        }
                        frame True {
                        }
                      }
                    }
                    frame #1 {
                      n256 = property on="Argument List Out" class="Arr (strict)"() -> ("Value"=w322:string[])  [unwired: 2 in, 2 out]
                      n257 = call "Set_Argument.vi"("Enable"=TRUE, "Argument"="run_started", "Argument List In"=w322) -> ("Argument List Out"=w323:string[])
                      n258 = property on="Argument List Out" class="Arr (strict)"("Value"=w323) -> ()  [unwired: 2 in, 2 out]
                    }
                  }
                }
              }
            }
          }
        }
        frame "End" {
        }
        frame "Idle" {
        }
      }
    }
  }
